vi "init.vi"(8 "error in (no error)":errorcluster, 10 "Inputs to Sine Wave":T1={"Frequency"=10.0, "Amplitude"=1.0, "Phase"=0.0, " Time"=0.0}, 11 "SineWave in":refnum<class "SineWave.lvclass">) -> (0 "error out":errorcluster, 3 "SineWave out":refnum<class "SineWave.lvclass">)   [LabVIEW 2015, in "SineWave.lvclass"]
uses:
  SineWave.lvclass
  Typedefs/PeriodicWaveInputs.ctl
  SineWave.lvclass/SineWave.ctl
  Typedefs/FAMTTypedefs.lvlib
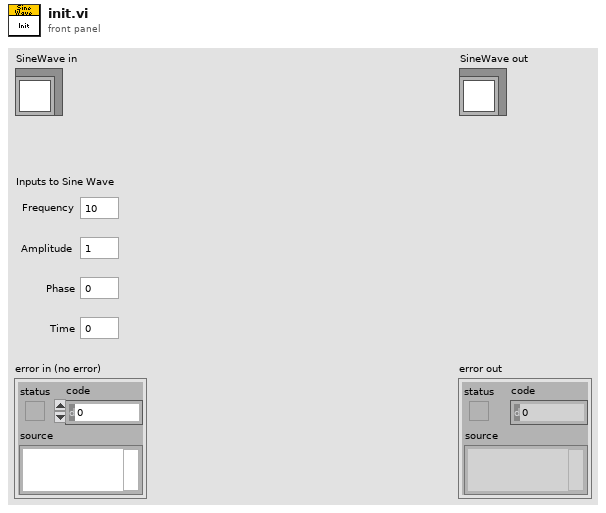
[diagram p1: front panel]
types:
  T1 = typedef "FAMTTypedefs.lvlib/PeriodicWaveInputs.ctl" = cluster{"Frequency":dbl, "Amplitude":dbl, "Phase":dbl, " Time":dbl}
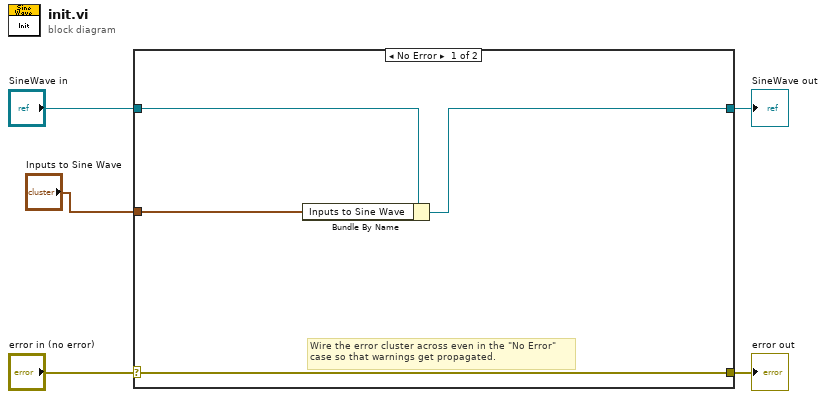
[diagram p0: block diagram]
diagram:
  n1 = case shown="No Error" "error in (no error)" {
    selector: "error in (no error)" -> [w9 w11]
    tunnel: [w9 w11] -> w4
    tunnel: [w6 w10] -> w2
    tunnel: "SineWave in" -> [w7 w10]
    tunnel: "Inputs to Sine Wave" -> [w8 _]
    frame No Error {
      # "Wire the error cluster across even in the \"No Error\"\ncase so that warnings get propagated."
      n2 = Bundle By Name(cluster=w7, "Inputs to Sine Wave"=w8) -> (w6:refnum<class "SineWave.lvclass">)
    }
    frame Error {
    }
  }
  "error out" <- w4
  "SineWave out" <- w2
